vi "Write Cache.vi"(8 "error in (no error)":errorcluster, 10 "Registry Cache in":u8[](array[numeric]), 11 "navX Registry Cache in":refnum<class "navX Registry Cache.lvclass">) -> (0 "error out":errorcluster, 3 "navX Registry Cache out":refnum<class "navX Registry Cache.lvclass">)   [LabVIEW 2015, in "navX Library v3.lvlib" / "navX Registry Cache.lvclass"]
uses:
  navX Registry Cache.lvclass
  navX Registry Cache.lvclass/navX Registry Cache.ctl
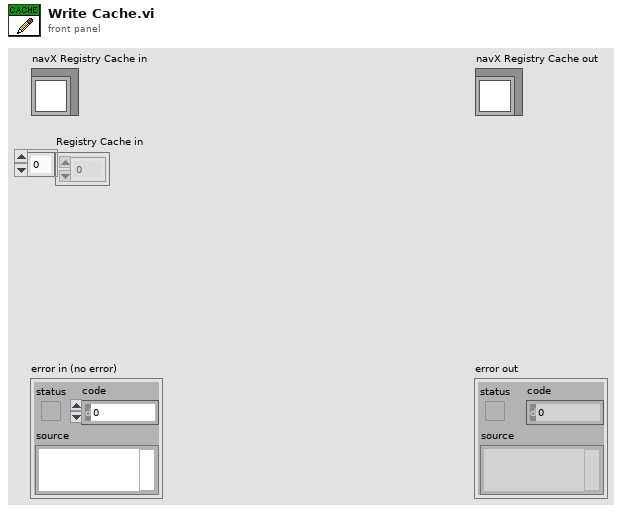
[diagram p1: front panel]
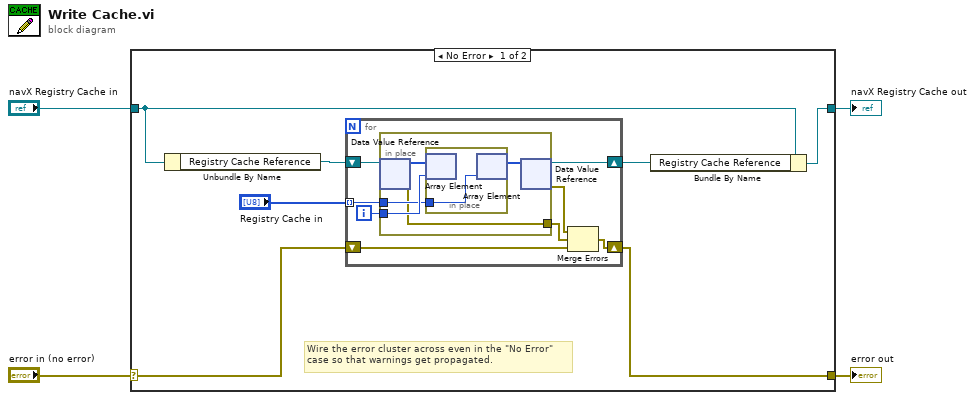
[diagram p0: block diagram]
diagram:
  n1 = case shown="No Error" "error in (no error)" {
    selector: "error in (no error)" -> [w6 w27]
    tunnel: [w5 w27] -> w3
    tunnel: [w9 w26] -> w1
    tunnel: "navX Registry Cache in" -> [w10 w26]
    frame No Error {
      # "Wire the error cluster across even in the \"No Error\"\ncase so that warnings get propagated."
      n2 = Unbundle By Name(w10) -> ("Registry Cache Reference"=w11:refnum<data-value>)
      n3 = for {
        tunnel: "Registry Cache in" -> [w17] mode=indexing
        shift-right: [w13] -> w5
        shift-left: w6 -> [w12]
        shift-right: [w18] -> w8
        shift-left: w11 -> [w19]
        i -> [w16]
        n4 = in-place {
          in-place-border: w17 -> [w21]
          in-place-border: w16 -> [w22]
          in-place-border: [w20] -> w14
          n5 = in-place-dvr #1(w19) -> (w24:u8[], w20:errorcluster)
          n6 = in-place {
            in-place-border: w21 -> [w25]
            n7 = in-place-array #2(w24, w22) -> ()  [unwired: 1 out]
            n8 = in-place-array #2(w25) -> (w23:u8[])  [unwired: 1 out]
          }
          n9 = in-place-dvr #1(w23) -> (w18:refnum<data-value>, w15:errorcluster)
        }
        n10 = Merge Errors(w15, w14, w12) -> (w13:errorcluster)
      }
      n11 = Bundle By Name(cluster=w10, "Registry Cache Reference"=w8) -> (w9:refnum<class "navX Registry Cache.lvclass">)
    }
    frame Error {
    }
  }
  "error out" <- w3
  "navX Registry Cache out" <- w1
